vi "Send Redraw Configuration.vi"(8 "error in (no error)":errorcluster, 11 "AssertEngine in":refnum<class "AssertEngine.lvclass">) -> (0 "error out":errorcluster)   [LabVIEW 2016, in "AssertEngine.lvlib" / "AssertEngine.lvclass"]
doc: "Sends the command to the user interface to redraw the parameters and assert data"
uses:
  AssertEngine.lvclass
  AssertEngine.lvclass/AssertEngine.ctl
  Log Assert/Assert Data.ctl
  UserInterface/UserInterface Messages/Draw Assert Data Msg/Draw Assert Data Msg.lvclass/Draw Assert Data Msg.ctl
  <vilib>/ActorFramework/Message Enqueuer/Message Enqueuer.lvclass/Message Enqueuer.ctl
  <vilib>/ActorFramework/Message Enqueuer/Enqueue.vi
  UserInterface/UserInterface Messages/Draw Assert Data Msg/Draw Assert Data Msg.lvclass
  C:/Program Files/National Instruments/LabVIEW 2016/vi.lib/ActorFramework/Message/Message.lvclass
  <vilib>/ActorFramework/Message Priority Queue/Priority Enqueue.vi
  AssertEngine.lvlib
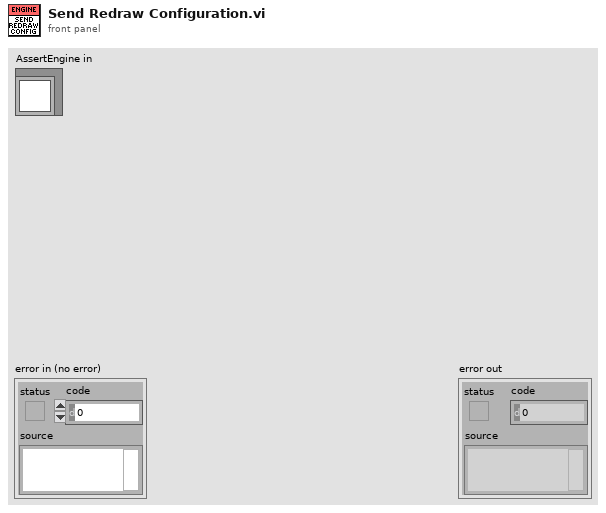
[diagram p1: front panel]
types:
  T1 = typedef "AssertEngine.lvlib/Assert Data.ctl" = cluster{"Assert Name":string, "Status":string, "Comment":string, "Eval String":string, "Failure Action":string, "Calling VI Name":string, "Assert VI Name":string, "Data Value":variant, "Assert VI UID":i32, "Assert Builder":string, "Build Timestamp":timestamp, "Last Update":timestamp, "Top Level VI Name":string, "Data Type":string}
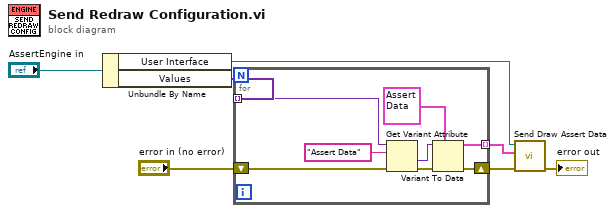
[diagram p0: block diagram]
diagram:
  n1 = Unbundle By Name("AssertEngine in") -> ("User Interface"=w5:refnum<class "Message Enqueuer.lvclass">, "Values"=w4:variant[])
  n2 = for {
    tunnel: w4 -> [w15] mode=indexing
    shift-right: [w9] -> w2
    shift-left: "error in (no error)" -> [w13]
    tunnel: [w8] -> w1 mode=indexing
    n3 = Get Variant Attribute(Variant=w15, name="Assert Data", error in=w13) -> (value=w11:variant, error out=w12:errorcluster)  [unwired: 1 in, 2 out]
    n4 = Variant To Data(error in=w12, type=T1 {"Assert Name"="", "Status"="", "Comment"="", "Eval String"="", "Failure Action"="", "Calling VI Name"="", "Assert VI Name"="", "Data Value"=variant, "Assert VI UID"=0, "Assert Builder"="", "Build Timestamp"=timestamp(0 s since 1904-01-01), "Last Update"=timestamp(0 s since 1904-01-01), "Top Level VI Name"="", "Data Type"=""} ("name"), Variant=w11) -> (data=w8:T1, error out=w9:errorcluster)
  }
  n5 = call "Send Draw Assert Data.vi"("error in (no error)"=w2, "Assert Array"=w1, "Message Enqueuer"=w5) -> ("error out"=→"error out":errorcluster)  [unwired: 7 in, 1 out]
